vi "readme.vi"() -> ()   [LabVIEW 2020]
doc: "A manual for the ORM library in the form of a VI. Open the VI and read the text on the block diagram."
uses:
  <vilib>/Viviota/shared/ORM_DBC_Mssql.lvlibp/SQL Connect.vi
  ORM_API/ORM_API.lvlib
  <vilib>/Viviota/shared/ORM_DBC_Mssql.lvlibp/DBC.lvclass
panel:
  in  "String":string="Please see \"Primary Example\" VI for a full implementation / description.\nBelow is additional/detailed information about how this system works.\n\nDOCUMENTATION FOR THE ORM LIBRARY\n\nThis library facilitates the connection between LabVIEW objects and database tables.  Currently, it supports the following database types:\n\n        SQLite\n        SQL Server (and SQL Server Express)\n        mySQL\n        postgreSQL\n        ODBC connections\n\n        (limited support with kdb+)\n\nThe library supports two different APIs a high level \"CRUD\" API (Create,Read,Update,Delete) that require minimal use of actual SQL calls.  And then a lower-level Query/Execute VI, which allows the user to provie explicit SQL statements.\n\nThis document describes the minimum that you must know in order to use both the low-level and CRUD capabilities of the library.\n\nFIRST STEP - DATABASE CONNECTION STRINGS\n\nYou must formulate a valid connection string for whichever database type you choose.  The sample connection strings presented\nhere have been tested and are valid.  They are not the only one possible, however.\n\nSQL Server:\n\nA valid connection string is ...\n\nData Source=SQLEXPRESS;Initial Catalog=DATABASE;Persist Security Info=false;Integrated Security=true; \n\nIn the above string,\n        Data Source = the name of the database server\n        Initial Catalog = the name of the database you will be using\n\npostgreSQL:\n\nA valid connection string is ...\n\nServer = localhost; Port = 5432; Database = database; User Id = postgres; Password = password;\n\nIn the above string, \n        Server = the name of the database server\n        Port = port used to access the server (5432 is the default port)\n        Database = the name of the database to be accessed\n        User Id = username to log in with; \"postgres\" is a default user name\n        Password = password for the same account\n\nSQLite:\n\nA valid connection string is ...\n\nData Source=c:\\projects\\mydb.db;Version=3;datetimeformat=CurrentCulture\n\nIn the above string,\n        Data Source = path to the database file\n        Version = major version of SQLite (currently 3)\n\nmySQL:\n\nA valid connection string is ...\n\nServer=localhost; Database=classicmodels; Uid=root; Pwd=password;\n\nIn the above string,\n        Server = name of the server hosting the DBMS\n        Database = name of the database\n        Uid = username for login\n        Pwd = password for login\n\nSECOND STEP - CREATE A DATABASE CONNECTION\n\nThere are two ways to connect.\n1. there is a poly VI which has an option for each database\n2. there is a \"Dynamic\" VI which uses a string/combo box to select the database type, and then instantiates the class dynamically.\n\nThis second interface exists because each database connection type is in it's own library, and this allows us to ONLY load the library (and dependencies) necessary.  This is very useful for building EXEs so that only the needed database types are kept around.\n\nIn addition to the database type (SQLite, PostgreSQL, etc) the \"connection\" VIs also require an interface provider.  Currently two providers are supported, ADO.NET and Dapper (also .NET) the Dapper interface is only maintained for legacy applications, and generally the ADO.NET provider is recommended\n\nTHIRD STEP - EXECUTE A DATABASE STATEMENT\n\nYou can use one of the following VI's from the palette to perform a query:\n\nQueryFirst_SQL.vim\n    returns the first row from your query, no matter how many rows were actually returned.\n\nQuery_SQL.vim\n    returns the full contents of your query, with help from one of the following VI's ...\n\n -  ToArray.vim\n -  Next.vim\n\nYou can use the following VI to perform other database functions.  It returns only the number of rows affected, so it is not really suitable for returning query results.\n\nExecute_SQL.vim\n\nin addition to the VIM versions which allow the results to be type cast into the target classes, there are static .VI versions of these VIs as well\n\nCRUD - INTRODUCTION\n\nCRUD stands for Create Read Update Delete.  These are the four basic operations that are done on data in a database.  In particular,\n    CREATE - refers to adding a row or rows to an existing database table using an Insert statement\n    READ - refers to querying or reading existing data in a table using a Select statement\n    UPDATE - refers to modifying an existing row or rows in a table using an Update statement\n    DELETE - refers to removing an existing row or rows from a table using a Delete statement\n\nEach of these functions is implemented in a VI and VIM of the same name.\nAdditionally there are three additional functions:\n     Bulk Create -- Allows the creation of multiple rows in a single command\n     Read All -- Allows the return of multiple rows\n     Read All Advanced -- Provides additional functionality for limits, offsets, and sortby conditions\n\n\nORM MAPPING\n\nThe mapping between table and class is done in one of two ways:\n1.  Through an explicit \"TypeMap\" class\n2.  Through the \"ObjectMap\" interface.\n\nTYPEMAP CLASS\nThis is a remnant from the original implementation (in 2018) before interfaces existed.\nFor each \"Data class\" that you want to associate with a database table, you need a \"data mapper\" class that inherits from the \"TypeMap\" class. \n\nAs an example data class, consider the class BB Players (baseball players).  The private data for this class is ...\n\n    pNum (I32) - not the players number on his uniform, just an identifier\n    pName(STR) - the player's name\n    pGames(I32) - the number of games played\n    pAverage(DBL) - the player's batting average\n    pAvailable(BOOL) - player is available for the next game or not\n\nThe corresponding table (SQL Server in this case) is ...\n\n    playerNum (int, not null, primary key)\n    name (varchar(50) null)\n    numGames (int, null)\n    average (float, null)\n    available (char(1), null)\n\nThe orders of the variables in the private data and the columns in the table match, but they don't have to.  Notice also that the LabVIEW boolean variable is represented by a char(1) column, for which the value will be 'Y' or 'N' (could also be 'T' or 'F').  This is a standard way (but not the only way) to handle a boolean value in SQL Server.  Note that the column names and LabVIEW variable names do not have to match.\n\nThe primary key column, playerNum in this example, should also be set as an IDENTITY.  This means that the database itself will generate a new value when a row is inserted.  Part of the work that the CRUD routines do is to \"grab\" that value and use it in the log table to help identify the row that was inserted.\n\nNOTE REGARDING postgreSQL:  You can create table and column names in mixed case in postgreSQL, but because incoming commands are all converted to lower case, you will be better off to keep ALL your postgreSQL table names and column names as lower case right from the beginning.\n\n\nA second class must be created that is associated specifically with your \"data\" class (described above).  The name of the class should reflect the fact that it is associated with the other class.  This class must inherit from the  the TypeMap class.  It has no private data of its own, but there is private data associated with the parent classes which will be used to associate your original data class to a particular table.\n\nThe only two overrides that MUST be created are the From LabVIEW and To LabVIEW methods.  These methods provide the \"glue\" that associates your data class with the database table.  It is where type conversions, if necessary, can be implemented to ensure that the LabVIEW types and the database types are compatible.\n\n\"From LabVIEW\" takes in the \"data\" class's data as a variant and outputs it as a DbRow.  A DbRow is essentially a dictionary that expresses a row of the associated table as a (name : value) pair.  The \"name\" is the column name in the table, and the \"value\" is its value taken from the input class data.  The dictionary is implemented in LabVIEW as an empty variant with an attribute associated with each (name : value) pair in the dictionary.\n\n\"To LabVIEW\" reverses this process, taking in DbRow data and putting it back into class data (as a variant).\n\n\nOBJECTMAP Interface\nAlternatively, you can add the ObjectMap.lvclass interface to your data class directly.  This will then have two overrides \"OM_FromLabVIEW\" and \"OM_ToLabVIEW\" that act in the exact same way as the To/From LabVIEW classes above.  However, in this case there's less overhead, since you don't need a completely separate class.\n\n\nUSING THE CLASS MAPPING\nThe classes above tell the system how to map data, but there is additional information required.  This is done using \"SetTypeMap.vi\"  This allows the association of a Data class with a Type Map (and meta information), that gets stored at the application level -- alternatively each CRUD / low-level VI also can take an explicit TypeMap input.\n\nIf using the 2 class method (a type map inheriting from the TypeMap Class) then you can provide that as input (along with the class of interest) to this VI.\n\nIf using the ObjectMap Interface method, you can specify just the generic TypeMap Class.\n\nIn either case, befor the class is provided, two Accessors MUST be specified: the \"Autokey\" and the \"Table Name\" properties.  The \"Autokey\" tells the system which value should be interpretted as the unique integer key of the table.  The \"Table Name\" specifies which table should be used for the class data storage/retrieval.\n\n\n\nTHE LOG MAP\nIn the base toolkit, there is a LogMap class that inherits from the TypeMap class.  If you decide to use this class as a mapper instead, whenever a \"Write\" action is performed (Create, Update, Delete) the action will also be logged in a table in the database (if the property \"LogTableName\" is specified)\n\nThe table associated with the data map class should be named \"Log\" and constructed as follows:\n\n    id (int, primary key, not null)\n    ActionTime (datetime)\n    ActionType (string)\n    ObjectTable (string)\n    ObjectID (int)\n    ObjectRepr (string)\n    Username (string)\n    Domain (string)\n    IP (string)\n    MachineGuid (string)\n\nThe above data types are for SQLite.  If you are using postgreSQL, note the following:\n\n    the table should be named \"log\" (all lower case)\n    all column names should be completely in lower case\n    actiontime type should be \"timestamp without time zone\"\n    string types shown above should be \"character varying\" with sufficient width specified (200 is plenty)\n\nFor mySQL, note the following:\n\n    use \"log\" for the table name (all lower case) - provided mySQL is in the default Windows configuration.\n    for the ActionTime column, the data type DateTime(6) works (it has been tested)\n    the ObjectRepr column can contain quite a bit of text; varchar(200) works for all database types"
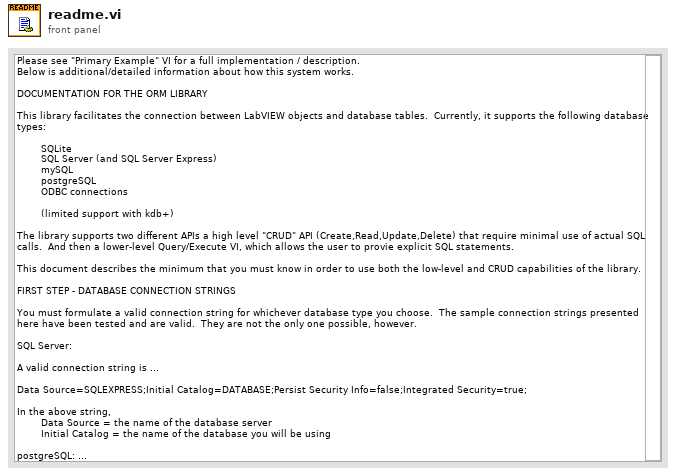
[diagram p1: front panel]
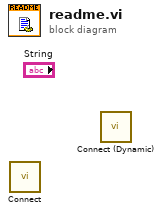
[diagram p0: block diagram]
diagram:
  n1 = call-poly "Connect.vi"() -> ()  [unwired: 10 in, 2 out]
  n2 = call "Connect (Dynamic).vi"() -> ()  [unwired: 10 in, 2 out]
